vi "Open.vi"(8 "error in (no error)":errorcluster, 10 "Send \"Connect client\"":bool, 11 "RP Communicator in":refnum<class "RP Communicator.lvclass">) -> (0 "error out":errorcluster, 3 "RP Communicator out":refnum<class "RP Communicator.lvclass">)   [LabVIEW 2016, in "RP Communicator.lvclass"]
uses:
  RP Communicator.lvclass
  RP Communicator.lvclass/RP Communicator.ctl
  RP Command.ctl
  RP Write Command TCP.vi
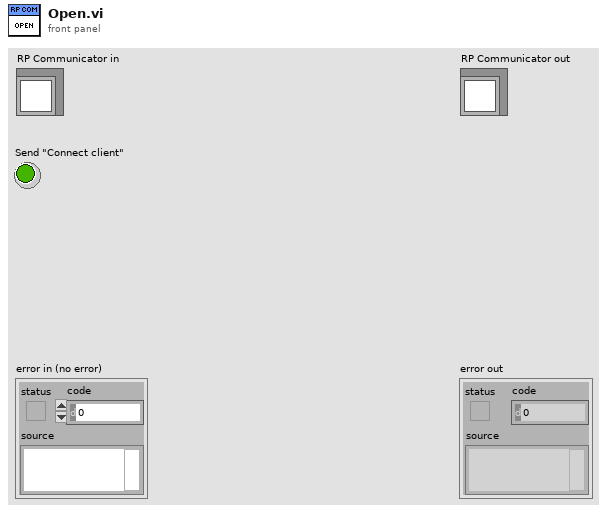
[diagram p1: front panel]
types:
  T1 = typedef "RP Command.ctl" = enum16{"Reset", "Read IDN", "Stop server", "Get status", "Get temperature", "Connect client", "Arm", "Software trigger", "Get whole buffer", "Get chunk", "System call", "Get config", "Set config", "Recieve data", "Recieve Calibartion", "Transmit data"}
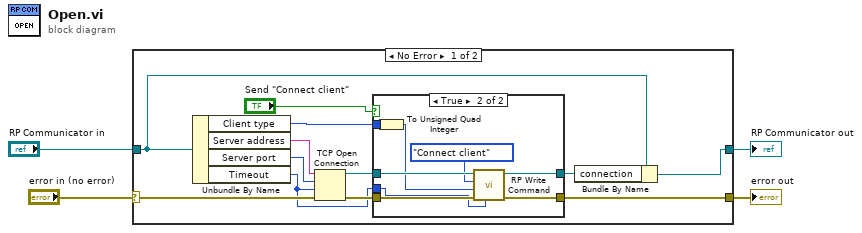
[diagram p0: block diagram]
diagram:
  n1 = case shown="No Error" "error in (no error)" {
    selector: "error in (no error)" -> [w14 w28]
    tunnel: [w7 w28] -> w3
    tunnel: [w9 w27] -> w1
    tunnel: "RP Communicator in" -> [w10 w27]
    frame No Error {
      n2 = Unbundle By Name(w10) -> ("Client type"=w11:enum16{"Control", "Reciever", "Transmitter"}, "Server address"=w16:string, "Server port"=w15:u16, "Timeout"=w5:i32)
      n3 = TCP Open Connection(address=w16, remote port or service name=w15, timeout ms (60000)=w5, error in (no error)=w14) -> (connection ID=w12:refnum<k5>, error out=w13:errorcluster)  [unwired: 1 in]
      n4 = case shown="True" "Send \"Connect client\"" {
        tunnel: w13 -> [w17 w26]
        tunnel: w12 -> [w18 w25]
        tunnel: w11 -> [_ w23]
        tunnel: [w18 w21] -> w8
        tunnel: [w17 w20] -> w7
        tunnel: w5 -> [_ w19]
        frame False {
        }
        frame True {
          n5 = To Unsigned Quad Integer(1:w23) -> (0:w22:u64)
          n6 = call-poly "RP Write Command.vi"("timeout ms (25000)"=w19, "Error In"=w26, "Command payload"=w22, "Command number"=RP_Command."Connect client", "connection ID"=w25) -> ("Error Out"=w20:errorcluster, "connection ID out"=w21:refnum<k5>)  [unwired: 4 in, 1 out]
        }
      }
      n7 = Bundle By Name(cluster=w10, "connection"=w8) -> (w9:refnum<class "RP Communicator.lvclass">)
    }
    frame Error {
    }
  }
  "error out" <- w3
  "RP Communicator out" <- w1
